vi "Emballa_BDD_listeXML.vi"(8 "entrée d'erreur (pas d'erreur)":errorcluster) -> (0 "sortie d'erreur":errorcluster, 1 "Numérique":i32, 2 "filenames":string[](array[string]), 3 "repertoireConfigs":path)   [LabVIEW 2020]
uses:
  Modules/FS/60_FS_Controles/60_FS_SetGet.ctl
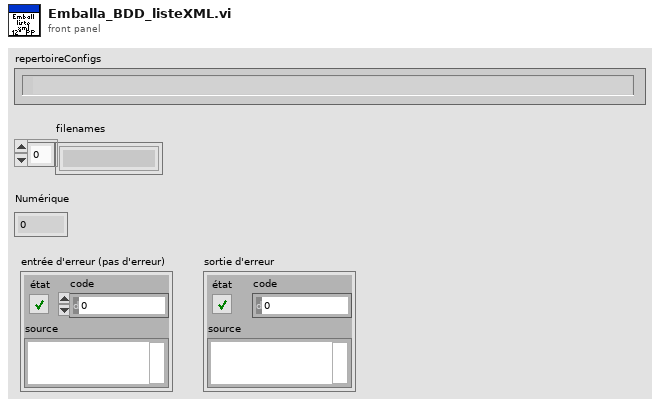
[diagram p1: front panel]
types:
  T1 = typedef "60_FS_SetGet.ctl" = enum16{"set", "get"}
  T2 = cluster{"Admin-réseau":path, "XML-Réseau":path, " Résultat tests-Réseau":path, " Archive prôbleme-Réseau":path, " Archive Test  Local":path}
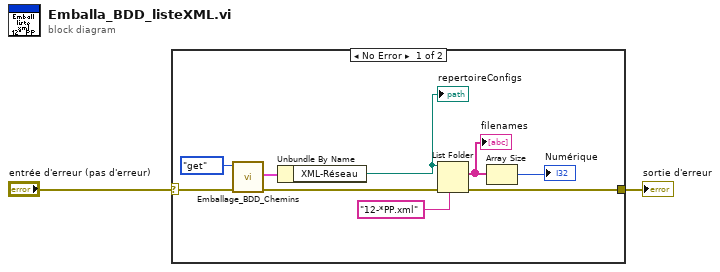
[diagram p0: block diagram]
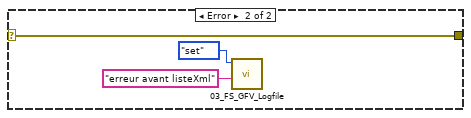
[diagram p2: hidden frame]
diagram:
  n1 = case shown="No Error" "entrée d'erreur (pas d'erreur)" {
    selector: "entrée d'erreur (pas d'erreur)" -> [w7 w14]
    tunnel: [w11 w14] -> w2
    frame No Error {
      n2 = call "Emballage_BDD_Chemins.vi"("error in (no error)"=w7, "SetGet"=60_FS_SetGet."get") -> ("error out"=w6:errorcluster, "CLT_Chemins_out"=w5:T2)  [unwired: 8 in]
      n3 = Unbundle By Name(w5) -> ("XML-Réseau"=w4:path)
      "repertoireConfigs" <- w4
      n4 = List Folder(path=w4, pattern="12-*PP.xml" ("filtre"), error in=w6) -> (filenames=w9:string[], error out=w11:errorcluster)  [unwired: 1 in, 2 out]
      "filenames" <- w9
      n5 = Array Size(array=w9) -> (size(s)=→"Numérique":i32)
    }
    frame Error {
      n6 = call "03_FS_GFV_Logfile.vi"("Chaîne"="erreur avant listeXml", "States"=60_FS_SetGet."set") -> ()  [unwired: 8 in, 2 out]
    }
  }
  "sortie d'erreur" <- w2
